vi "RecordingLoop.vi"(8 "error in (no error)":errorcluster, 10 "Data Queue In":refnum<queue>, 11 "State Queue":refnum<queue>) -> (0 "error out":errorcluster, 2 "Data Queue Out":refnum<queue>)   [LabVIEW 2017, in "ImageAcquisitionLibrary.lvlib"]
uses:
  ImageAcquisitionLibrary.lvlib
  RecordingState.ctl
  Acquisition/AcquireData.ctl
  RecordingData.ctl
  <vilib>/vision/Image Controls.llb/IMAQ Image.ctl
  <vilib>/vision/Avi.llb/IMAQ AVI2 Refnum.ctl
  Settings/Settings.ctl
  <vilib>/userdefined/High Color/IMAQdx.ctl
  Tracking/TrackingSettings.ctl
  Settings/Calibration.ctl
  <vilib>/Utility/error.llb/DialogType.ctl
  SettingsGlobal.vi
panel:
  in  "Recording Data 2":T1
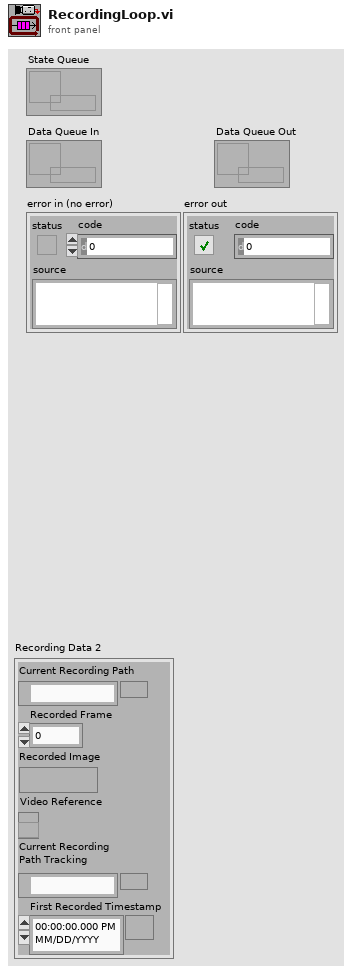
[diagram p1: front panel]
types:
  T1 = typedef "ImageAcquisitionLibrary.lvlib/RecordingData.ctl" = cluster{"Current Recording Path":path, "Recorded Frame":i32, "Recorded Image":T2, "Video Reference":T3, "Current Recording \nPath Tracking":path, "First Recorded Timestamp":timestamp}
  T2 = typedef "IMAQ Image.ctl" = refnum<image>
  T3 = typedef "IMAQ AVI2 Refnum.ctl" = refnum<k20>
  T4 = typedef "ImageAcquisitionLibrary.lvlib/Settings.ctl" = cluster{"Harware Configuration":cluster{"Camera":T5, "Frames Per Second":u32, "Simulate Recording":bool, "Simulated Recording Sample":path, "Timestamp Method":enum16{"System Timestamp", "Camera Timestamp", "IMAQdx Timestamp"}}, "Base Recording Path":path, "Type Of Recording":string, "Recording Codec":string, "TrackingSettings":T6, "Calibration":T8, "Broadcast Length":i32}
  T5 = typedef "IMAQdx.ctl" = refnum<k21>
  T6 = typedef "ImageAcquisitionLibrary.lvlib/TrackingSettings.ctl" = cluster{"Max Radius":i32, "Threshold":sgl, "ROI":T7}
  T7 = typedef "IMAQ Rectangle" = cluster{"Left":i32, "Top":i32, "Right":i32, "Bottom":i32, "Rotation":dbl}
  T8 = typedef "ImageAcquisitionLibrary.lvlib/Calibration.ctl" = cluster{"Pixel Width (X)":dbl, "Pixel Height (Y)":dbl}
  T9 = typedef "ImageAcquisitionLibrary.lvlib/RecordingState.ctl" = enum16{"Idle", "Start Recording", "Record", "Update Settings", "Stop Recording", "Exit"}
  T10 = typedef "ImageAcquisitionLibrary.lvlib/AcquireData.ctl" = cluster{"Frame Data":cluster{"Image":u32[][], "Timestamp":timestamp, "Image Type":T11, "Dropped Frames":u32}, "Tracking Data":cluster{"Positions":dbl[][], "Timestamp":timestamp}, "Tracked?":bool}
  T11 = typedef "Image Type" = u32
  T12 = typedef "DialogType.ctl" = u16
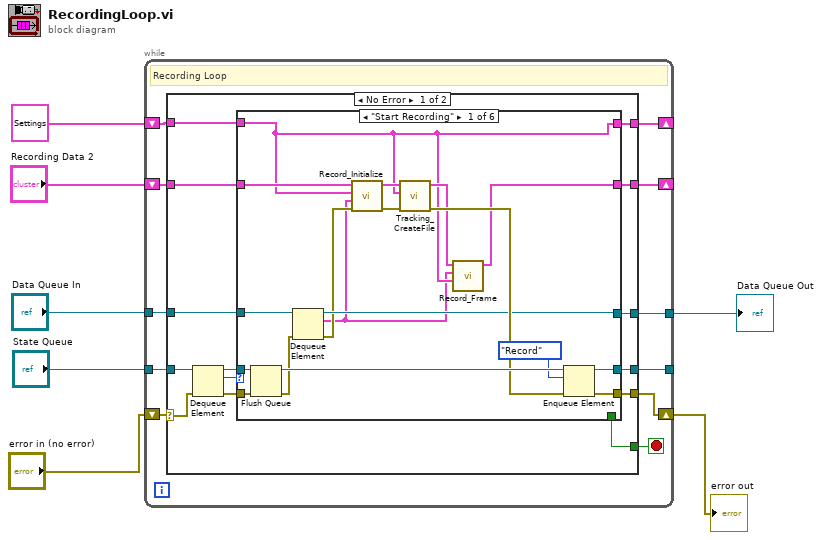
[diagram p0: block diagram]
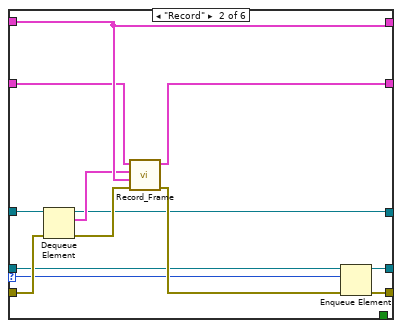
[diagram p2: hidden frame]
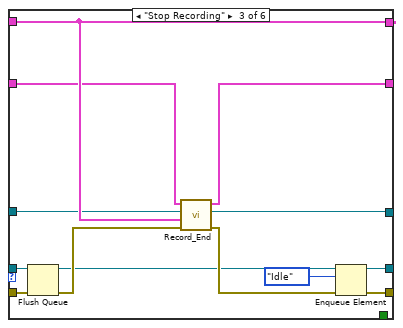
[diagram p3: hidden frame]
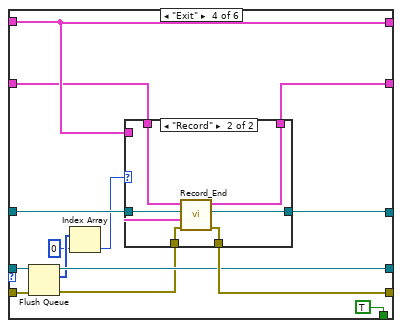
[diagram p4: hidden frame]
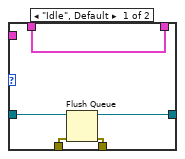
[diagram p5: hidden frame]
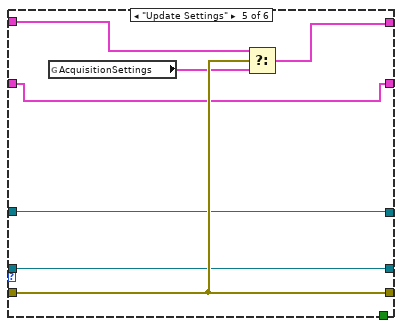
[diagram p6: hidden frame]
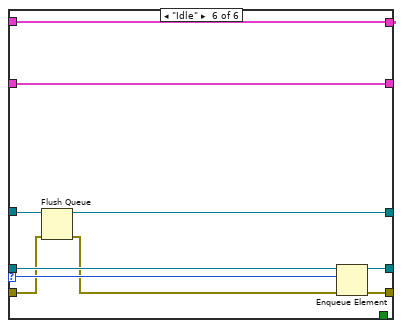
[diagram p7: hidden frame]
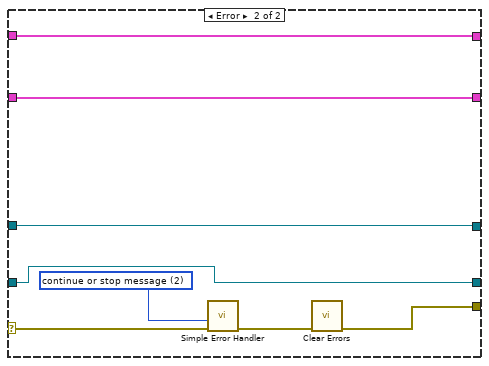
[diagram p8: hidden frame]
diagram:
  n1 = while {
    tunnel: "State Queue" -> [w14]
    shift-right: [w17] -> w5
    shift-left: "error in (no error)" -> [w13]
    shift-right: [w16] -> _
    shift-left: T4 {"Harware Configuration"={"Camera"="cam1", "Frames Per Second"=15, "Simulate Recording"=FALSE, "Simulated Recording Sample"=path "", "Timestamp Method"=enum."Camera Timestamp"}, "Base Recording Path"=path "", "Type Of Recording"="", "Recording Codec"="", "TrackingSettings"={"Max Radius"=0, "Threshold"=160.0, "ROI"={"Left"=0, "Top"=0, "Right"=0, "Bottom"=0, "Rotation"=0.0}}, "Calibration"={"Pixel Width (X)"=10.0, "Pixel Height (Y)"=100.0}, "Broadcast Length"=0} ("Settings") -> [w18]
    tunnel: "Data Queue In" -> [w12]
    tunnel: [w11] -> _
    shift-right: [w9] -> _
    shift-left: "Recording Data 2" -> [w10]
    tunnel: [w8] -> w1
    stop <- w15 stop-if-true
    # "Recording Loop"
    n2 = case shown="No Error" w13 {
      selector: w13 -> [w26 w126]
      tunnel: w18 -> [w32 w127]
      tunnel: [w31 w123] -> w17
      tunnel: [w30 w127] -> w16
      tunnel: [w29 _] -> w15
      tunnel: w14 -> [w27 w121]
      tunnel: [w28 w120] -> w9
      tunnel: w12 -> [w22 w122]
      tunnel: [w21 w121] -> w11
      tunnel: w10 -> [w20 w120]
      tunnel: [w19 w122] -> w8
      frame No Error {
        n3 = Dequeue Element(queue=w27, error in (no error)=w26) -> (queue out=w24:refnum<queue>, element=w23:T9, error out=w25:errorcluster)  [unwired: 1 in, 1 out]
        n4 = case shown="\"Start Recording\"" w23 {
          selector: w23 -> [_ w56 _ _ _ w115]
          tunnel: w32 -> [w34 w63 w73 w86 w109 w119]
          tunnel: w25 -> [w50 w62 w76 w88 w107 w113]
          tunnel: [w46 w58 w69 w90 w107 w118] -> w31
          tunnel: [w34 w63 w73 w86 w108 w119] -> w30
          tunnel: w24 -> [w49 w57 w74 w87 w103 w116]
          tunnel: [_ _ _ TRUE _ _] -> w29
          tunnel: [w35 w52 w64 w80 w105 w110] -> w28
          tunnel: w22 -> [w40 w60 w71 w85 w104 w114]
          tunnel: [w45 w55 w68 w83 w103 w117] -> w21
          tunnel: w20 -> [w41 w53 w72 w84 w105 w110]
          tunnel: [w39 w51 w65 w81 w104 w111] -> w19
          frame "Start Recording" {
            n5 = Flush Queue(queue=w49, error in (no error)=w50) -> (queue out=w44:refnum<queue>, error out=w38:errorcluster)  [unwired: 1 out]
            n6 = Dequeue Element(queue=w40, error in (no error)=w38) -> (queue out=w39:refnum<queue>, element=w33:T10, error out=w37:errorcluster)  [unwired: 1 in, 1 out]
            n7 = call "Record_Initialize.vi"("error in"=w37, "First Image in"=w33, "Settings in"=w34, "Recording Data"=w41) -> ("error out"=w48:errorcluster, "Recording Data Out"=w47:T1)  [unwired: 6 in]
            n8 = call "Tracking_CreateFile.vi"("error in"=w48, "Settings in"=w34, "Recording Data"=w47) -> ("error out"=w43:errorcluster, "Recording Data 2"=w36:T1)  [unwired: 7 in]
            n9 = call "Record_Frame.vi"("Settings"=w34, "Image Data"=w33, "Recording Data In"=w36) -> ("Recording Data Out"=w35:T1)  [unwired: 7 in, 1 out]
            n10 = Enqueue Element(queue=w44, element=RecordingState."Record", error in (no error)=w43) -> (queue out=w45:refnum<queue>, error out=w46:errorcluster)  [unwired: 1 in, 1 out]
          }
          frame "Record" {
            n11 = Dequeue Element(queue=w60, error in (no error)=w62) -> (queue out=w51:refnum<queue>, element=w54:T10, error out=w61:errorcluster)  [unwired: 1 in, 1 out]
            n12 = call "Record_Frame.vi"("error in"=w61, "Settings"=w63, "Image Data"=w54, "Recording Data In"=w53) -> ("error out"=w59:errorcluster, "Recording Data Out"=w52:T1)  [unwired: 6 in]
            n13 = Enqueue Element(queue=w57, element=w56, error in (no error)=w59) -> (queue out=w55:refnum<queue>, error out=w58:errorcluster)  [unwired: 1 in, 1 out]
          }
          frame "Stop Recording" {
            n14 = Flush Queue(queue=w74, error in (no error)=w76) -> (queue out=w67:refnum<queue>, error out=w75:errorcluster)  [unwired: 1 out]
            n15 = call "Record_End.vi"("error in"=w75, "Settings in"=w73, "Data Queue"=w71, "Recording Data"=w72) -> ("error out"=w70:errorcluster, "Data Queue Out"=w65:refnum<queue>, "Recording Data 2"=w64:T1)  [unwired: 5 in]
            n16 = Enqueue Element(queue=w67, element=RecordingState."Idle", error in (no error)=w70) -> (queue out=w68:refnum<queue>, error out=w69:errorcluster)  [unwired: 1 in, 1 out]
          }
          frame "Exit" {
            n17 = Flush Queue(queue=w87, error in (no error)=w88) -> (queue out=w83:refnum<queue>, remaining elements=w79:T9[], error out=w82:errorcluster)
            n18 = Index Array(array=w79, index=0) -> (element=w77:T9)
            n19 = case shown="\"Record\"" w77 {
              tunnel: [w94 w102] -> w90
              tunnel: w86 -> [_ w101]
              tunnel: w85 -> [w92 w100]
              tunnel: w84 -> [w95 w99]
              tunnel: w82 -> [w93 w98]
              tunnel: [w91 w97] -> w81
              tunnel: [w95 w96] -> w80
              frame "Idle", Default {
                n20 = Flush Queue(queue=w92, error in (no error)=w93) -> (queue out=w91:refnum<queue>, error out=w94:errorcluster)  [unwired: 1 out]
              }
              frame "Record" {
                n21 = call "Record_End.vi"("error in"=w98, "Settings in"=w101, "Data Queue"=w100, "Recording Data"=w99) -> ("error out"=w102:errorcluster, "Data Queue Out"=w97:refnum<queue>, "Recording Data 2"=w96:T1)  [unwired: 5 in]
              }
            }
          }
          frame "Update Settings" {
            n22 = global read "SettingsGlobal.vi" "AcquisitionSettings"() -> (w106:T4)
            n23 = Select(t=w109, s=w107, f=w106) -> (s? t:f=w108:T4)
          }
          frame "Idle" {
            n24 = Flush Queue(queue=w114, error in (no error)=w113) -> (queue out=w111:refnum<queue>, error out=w112:errorcluster)  [unwired: 1 out]
            n25 = Enqueue Element(queue=w116, element=w115, error in (no error)=w112) -> (queue out=w117:refnum<queue>, error out=w118:errorcluster)  [unwired: 1 in, 1 out]
          }
        }
      }
      frame Error {
        w125 = T12 2 items=["no dialog", "OK message", "continue or stop message", "OK message + warnings", "continue/stop + warnings"] ("type of dialog (OK msg:1)")
        n26 = call <vilib>:"Simple Error Handler.vi"("type of dialog (OK msg:1)"=w125, "error in (no error)"=w126) -> ("error out"=w124:errorcluster)  [unwired: 3 in, 4 out]
        n27 = call <vilib>:"Clear Errors.vi"("error in (no error)"=w124) -> ("error out"=w123:errorcluster)  [unwired: 5 in, 1 out]
      }
    }
  }
  "error out" <- w5
  "Data Queue Out" <- w1
